vi "Camera - Find Marker.vi"(9 "Minimum Match Score":sgl, 10 "marker template relative path":string="BowMarker.bmp", 11 "Image In":T2(plugin-control)) -> (0 "Marker found?":T1, 1 "Best Match Position":cluster{"x":sgl, "y":sgl}, 2 "Best Match Angle":sgl, 3 "Image Out":T2)   [LabVIEW 2011]
doc: "Finds a glyph in an image, and returns: a boolean of whether the glyph could be found, the location of the best match in the image, and its rotation from the glyph template.\n\nCoders: Gray, Jason and Cory"
uses:
  <vilib>/vision/Image Controls.llb/IMAQ Image.ctl
  2-RIO/2 Typedefs/indicator LED.ctl
  <vilib>/vision/NI_Vision_Development_Module.lvlib
panel:
  out "Best Match":T3
  out "glyph path":path
  out "Marker":T2(plugin-control)
  in  "Settings":T4={"Match Mode"=1, "Number of Matches Requested"=1, "Minimum Match Score"=800.0, "SubPixel Accuracy"=FALSE, "Rotation Angle Ranges"=[], "Show Search Area"=FALSE, "Show Result"=TRUE} {"Rotation Angle Ranges"."End" format="%.1f"; "Rotation Angle Ranges"."Start" format="%.1f"; "Minimum Match Score" min=0 max=1000 format="%.2f"; "Number of Matches Requested" min=1; "Match Mode" items=["Shift Invariant", "Rotation Invariant"]}
  out "Matches":T5(array[cluster]) {"Bounding Box"."y" format="%.2f"; "Bounding Box"."x" format="%.2f"; "Position"."y" format="%.2f"; "Position"."x" format="%.2f"; "Score" format="%.2f"; "Scale" format="%.2f"; "Angle" format="%.2f"}
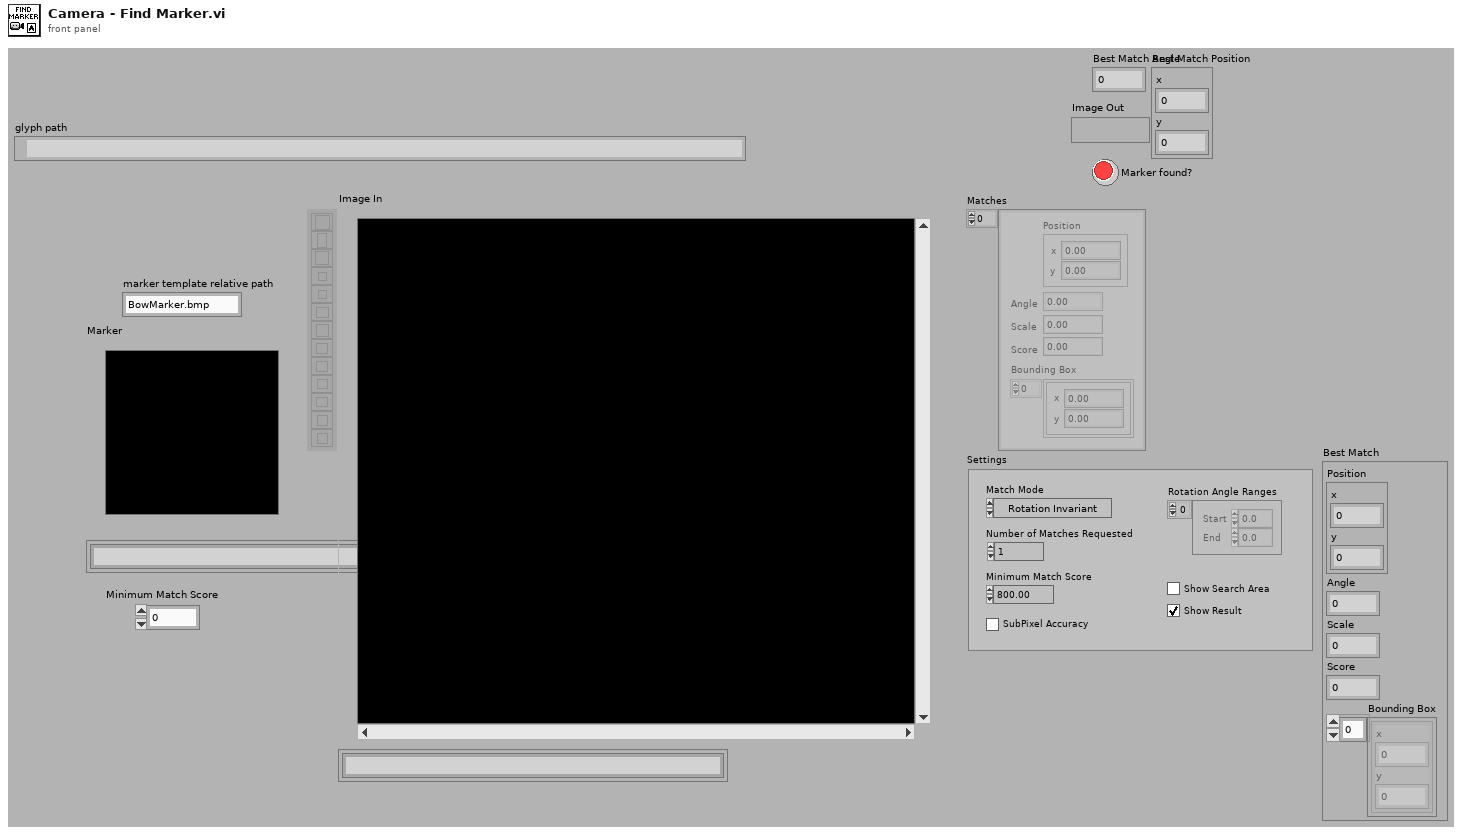
[diagram p1: front panel]
types:
  T1 = typedef "indicator LED.ctl" = bool
  T2 = typedef "IMAQ Image.ctl" = refnum<image>
  T3 = cluster{"Position":cluster{"x":sgl, "y":sgl}, "Angle":sgl, "Scale":sgl, "Score":sgl, "Bounding Box":cluster{"x":sgl, "y":sgl}[]}
  T4 = cluster{"Match Mode":u16, "Number of Matches Requested":i32, "Minimum Match Score":sgl, "SubPixel Accuracy":bool, "Rotation Angle Ranges":cluster{"Start":sgl, "End":sgl}[], "Show Search Area":bool, "Show Result":bool}
  T5 = cluster{"Position":cluster{"x":sgl, "y":sgl}, "Angle":sgl, "Scale":sgl, "Score":sgl, "Bounding Box":cluster{"x":sgl, "y":sgl}[]}[]
  T6 = typedef "Image Type" = u32
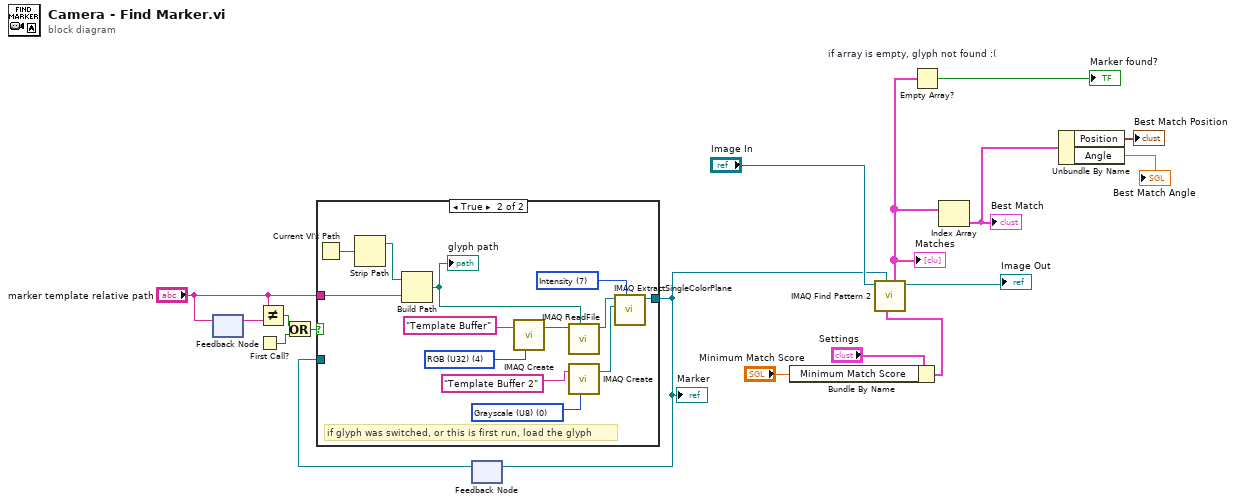
[diagram p0: block diagram]
diagram:
  n1 = feedback-in #1("marker template relative path") -> ()
  n2 = feedback #1() -> (w14:string)  [unwired: 1 in]
  n3 = First Call?() -> (First Call?: T/F=w9:bool)
  n4 = Not Equal?(x="marker template relative path", y=w14) -> (x != y?=w10:bool)
  n5 = Or(x=w10, y=w9) -> (x .or. y?=w11:bool)
  n6 = feedback #2() -> (w12:T2)  [unwired: 1 in]
  n7 = case shown="True" w11 {
    tunnel: [w18 w28] -> w13
    tunnel: "marker template relative path" -> [_ w19]
    tunnel: w12 -> [w18 _]
    frame False {
      # "if the path has not changed,\njust keep the same glyph from last time"
    }
    frame True {
      w25 = T6 0 items=["Grayscale (U8)", "Grayscale (I16)", "Grayscale (SGL)", "Complex (CSG)", "RGB (U32)", "HSL (U32)", "RGB (U64)", "Grayscale (U16)"] ("Image Type")
      w27 = 7 items=["Red", "Green", "Blue", "Hue", "Saturation", "Luminance", "Value", "Intensity"] ("Color Plane")
      w29 = T6 4 items=["Grayscale (U8)", "Grayscale (I16)", "Grayscale (SGL)", "Complex (CSG)", "RGB (U32)", "HSL (U32)", "RGB (U64)", "Grayscale (U16)"] ("Image Type")
      # "if glyph was switched, or this is first run, load the glyph"
      n8 = Current VI's Path() -> (path=w21:path)
      n9 = Strip Path(path=w21) -> (stripped path=w20:path)  [unwired: 1 out]
      n10 = Build Path(base path=w20, name or relative path=w19) -> (appended path=w22:path)
      "glyph path" <- w22
      n11 = call "IMAQ Create"("Image Name"="Template Buffer", "Image Type"=w29) -> ("New Image"=w30:T2)  [unwired: 3 in, 1 out]
      n12 = call "IMAQ ReadFile"("File Path"=w22, "Image"=w30) -> ("Image Out"=w24:T2)  [unwired: 5 in, 4 out]
      n13 = call "IMAQ Create"("Image Name"="Template Buffer 2", "Image Type"=w25) -> ("New Image"=w23:T2)  [unwired: 3 in, 1 out]
      n14 = call "IMAQ ExtractSingleColorPlane"("Color Plane"=w27, "Image Dst"=w23, "Image Src"=w24) -> ("Image Dst Out"=w28:T2)  [unwired: 7 in, 1 out]
    }
  }
  "Marker" <- w13
  n15 = feedback-in #2(w13) -> ()
  n16 = Bundle By Name(cluster="Settings", "Minimum Match Score"="Minimum Match Score") -> (w2:T4)
  n17 = call "IMAQ Find Pattern 2"("Settings"=w2, "Template"=w13, "Image"="Image In") -> ("Image Out"=→"Image Out":T2, "Matches"=w5:T5)  [unwired: 3 in, 4 out]
  "Matches" <- w5
  n18 = Empty Array? "if array is empty, glyph not found :("(array=w5) -> (empty?=→"Marker found?":bool)
  n19 = Index Array(array=w5) -> (element=w8:T3)  [unwired: 1 in]
  "Best Match" <- w8
  n20 = Unbundle By Name(w8) -> ("Position"=→"Best Match Position":cluster{"x":sgl, "y":sgl}, "Angle"=→"Best Match Angle":sgl)
